vi "get_data_for_this_device.vi"(8 "error in (no error)":errorcluster, 11 "DAQmxWriteSignals in":refnum<class "SignalWriterMM140725DAQmx.lvclass">) -> (0 "error out":errorcluster, 2 "data":dbl[][](array[numeric]), 3 "DAQmxWriteSignals out":refnum<class "SignalWriterMM140725DAQmx.lvclass">)   [LabVIEW 2010, in "SignalWriterMM140725DAQmx.lvclass"]
uses:
  SignalWriterMM140725DAQmx.lvclass
  common/enumerations/functional_global_action_enum.ctl
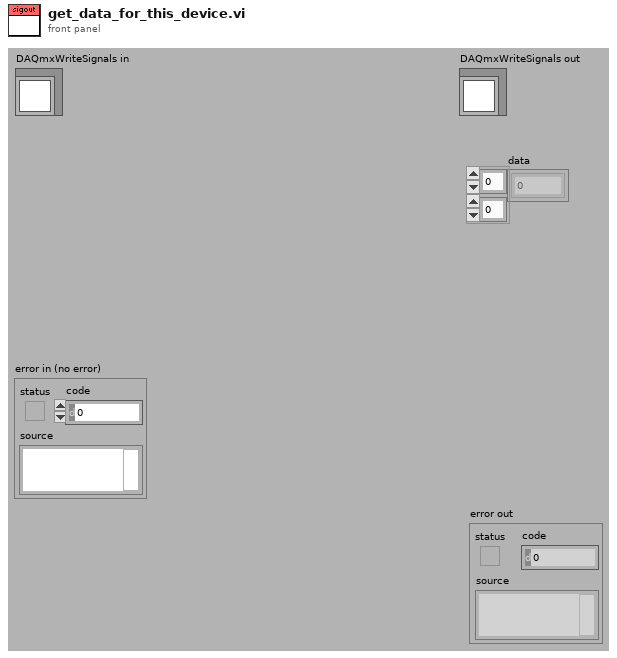
[diagram p1: front panel]
types:
  T1 = typedef "functional_global_action_enum.ctl" = enum16{"get", "set", "reset"}
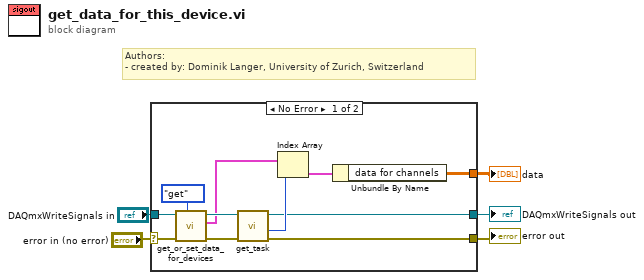
[diagram p0: block diagram]
diagram:
  # "Authors: \n- created by: Dominik Langer, University of Zurich, Switzerland"
  n1 = case shown="No Error" "error in (no error)" {
    selector: "error in (no error)" -> [w14 w18]
    tunnel: [w7 w18] -> w4
    tunnel: [w8 w17] -> w3
    tunnel: "DAQmxWriteSignals in" -> [w12 w17]
    tunnel: [w6 _] -> w5
    frame No Error {
      n2 = call-dynamic "get_or_set_data_for_devices.vi"("action"=functional_global_action_enum."get", "error in (no error)"=w14, "DAQmxWriteSignals in"=w12) -> ("error out"=w13:errorcluster, "data for devices out"=w10:cluster{"data for channels":dbl[][]}[], "DAQmxWriteSignals out"=w11:refnum<class "SignalWriterMM140725DAQmx.lvclass">)  [unwired: 1 in, 5 out]
      n3 = call-dynamic "get_task.vi"("error in (no error)"=w13, "DAQmxWriteSignals in"=w11) -> ("error out"=w7:errorcluster, "index"=w16:i32, "DAQmxWriteSignals out"=w8:refnum<class "SignalWriterMM140725DAQmx.lvclass">)  [unwired: 7 out]
      n4 = Index Array(array=w10, index=w16) -> (element=w15:cluster{"data for channels":dbl[][]})
      n5 = Unbundle By Name(w15) -> ("data for channels"=w6:dbl[][])
    }
    frame Error {
    }
  }
  "error out" <- w4
  "DAQmxWriteSignals out" <- w3
  "data" <- w5
